vi "Convert Assert Event Data to Test Case - Error (ERR) with Call Chain - Stack Trace contains Call Chain.vi"() -> ()   [LabVIEW 2013, in "JUnit Conversion Tests.lvlib"]
uses:
  <vilib>/addons/_JKI Toolkits/Caraya/classes/Test Result/Assert Event Data (Extended).ctl
  JUnit XML/Test Case/Test Case.lvclass/Test Case.ctl
  JUnit XML/Test Case/Read Stack Trace.vi
  <vilib>/addons/_JKI Toolkits/Caraya/classes/Assert/Assert Equal Value_Variant.vi
  JUnit Conversion Tests.lvlib
  JUnit Conversion/JUnit Conversion.lvlib
  <vilib>/addons/_JKI Toolkits/Caraya/classes/Test Result/Test Result.lvclass
  <vilib>/addons/_JKI Toolkits/Caraya/classes/Assert/Assert.lvclass
  <vilib>/addons/_JKI Toolkits/Caraya/classes/Test/Test.lvclass
  JUnit XML/Test Case/Test Case.lvclass
panel:
  out "error out":errorcluster
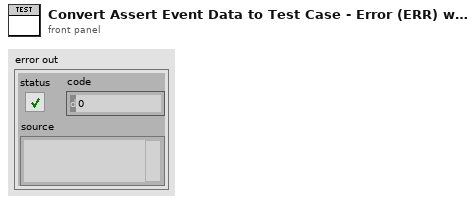
[diagram p1: front panel]
types:
  T1 = typedef "Caraya.lvlib/Test Result.lvclass/Assert Event Data (Extended).ctl" = cluster{"name":string, "passed":bool, "call-chain":string[], "test-error":errorcluster, "timestamp":timestamp, "assert-id":string, "test-id":string, "time":dbl, "message":string, "properties":variant, "measurements":variant, "user-defined":variant}
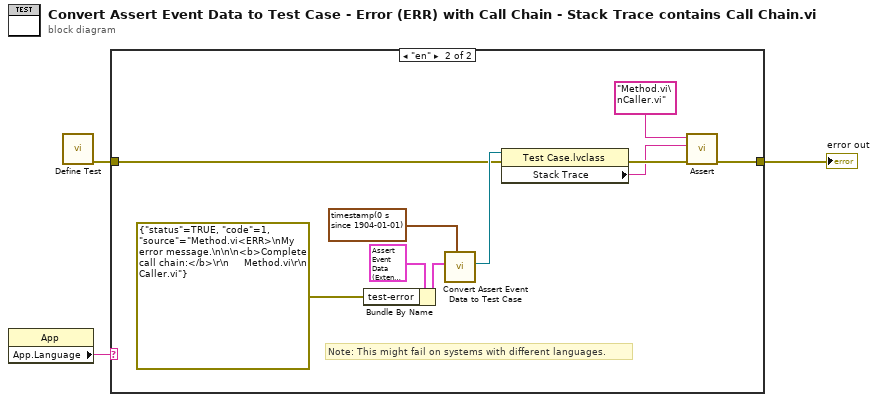
[diagram p0: block diagram]
diagram:
  n1 = property class="App"() -> ("App.Language"=w2:string)  [unwired: 2 in, 2 out]
  n2 = call <vilib>:"Define Test.vi"() -> ("error out"=w1:errorcluster)  [unwired: 10 in, 1 out]
  n3 = case shown="\"en\"" w2 {
    tunnel: [w4 w8] -> w3
    tunnel: w1 -> [w4 w5]
    frame Default {
    }
    frame "en" {
      # "Note: This might fail on systems with different languages."
      n4 = Bundle By Name(cluster=T1 {"name"="", "passed"=FALSE, "call-chain"=[], "test-error"={"status"=FALSE, "code"=0, "source"=""}, "timestamp"=timestamp(0 s since 1904-01-01), "assert-id"="", "test-id"="", "time"=-1.0, "message"="", "properties"=variant, "measurements"=variant, "user-defined"=variant} ("Assert Event Data"), "test-error"=errorcluster {"status"=TRUE, "code"=1, "source"="Method.vi<ERR>\nMy error message.\n\n\n<b>Complete call chain:</b>\r\n     Method.vi\r\n     Caller.vi"} ("error out")) -> (w13:T1)
      n5 = call "Convert Assert Event Data to Test Case.vi"("Start Time"=timestamp(0 s since 1904-01-01), "Assert Event Data"=w13) -> ("Test Case"=w12:refnum<class "Test Case.lvclass">)  [unwired: 9 in]
      n6 = property class="Test Case.lvclass"(reference=w12, error in=w5) -> (error out=w11:errorcluster, "Stack Trace"=w10:string)  [unwired: 1 out]
      n7 = call-poly <vilib>:"Assert.vi"("error in (no error)"=w11, "Y"=w10, "X"="Method.vi\nCaller.vi" ("message")) -> ("error out"=w8:errorcluster)  [unwired: 7 in, 1 out]
    }
  }
  "error out" <- w3
